vi "FPGAcode4_Test3.vi"() -> ()   [LabVIEW 2015]
uses:
  Limits_In.ctl
  Detector_Cluster.ctl
  <vilib>/Platform/TimedLoop/XDataNode/timing_clust.ctl
  <vilib>/Platform/TimedLoop/XDataNode/nitl_modes.ctl
  <vilib>/Platform/TimedLoop/XDataNode/wakeup.ctl
  Correlations.ctl
  <vilib>/rvi/Emulation/niFpgaGetClockAttributes.vi
  <vilib>/rvi/Emulation/niFpgaSctlEmulationGetInTimedLoop.vi
  <vilib>/rvi/Emulation/niFpgaEmulationReportErrorSimple.vi
  <vilib>/rvi/Emulation/niFpgaProcessEmulError.vi
  <vilib>/rvi/eio/common/nirviEmuTemplateMethod_errors.vi
  <vilib>/rvi/Emulation/niFpgaCriticalErrorInLSC.vi
  <vilib>/eio/EIONode/EIONode.xnode
  <vilib>/Platform/TimedLoop/XDataNode/XDataNode.xnode
  <vilib>/Platform/TimedLoop/XDataNode/XDNodeRunTimeDep.lvlib
panel:
  out "Detectors":T1
  in  "User Trigger?":bool
  in  "User Trigger Distance":fxp<+/-,34,18> format="%.3g"
  out "User Trigger":bool
  in  "Charge Error Factor":fxp<+,32,0>=0.19999999995343387 format="%_2g"
  in  "Threshold Factor":fxp<+/-,32,16>=1.149993896484375 format="%.2g"
  out "DCS 2":bool
  out "DCS 1":bool
  in  "Limits":T2={"High Charge Limit"=4.54747350780585e-13, "Low Charge Limit"=0.0, "High Velocity Limit"=262143.0, "Low Velocity Limit"=0.0, "High Mass Limit"=7.27595761248936e-12, "Low Mass Limit"=0.0, "High Voltage"=2200000.0}
  in  "Calibrate":bool=TRUE
  in  "Armed":bool
  out "Plates":bool
  in  "One Shot":bool
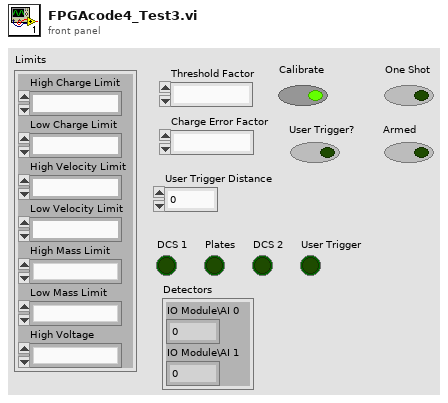
[diagram p1: front panel]
types:
  T1 = cluster{"IO Module\\AI 0":i16, "IO Module\\AI 1":i16}
  T2 = typedef "Limits_In.ctl" = cluster{"High Charge Limit":fxp<+,32,-41>, "Low Charge Limit":fxp<+,32,-41>, "High Velocity Limit":fxp<+,18,18>, "Low Velocity Limit":fxp<+,18,18>, "High Mass Limit":fxp<+/-,33,-36>, "Low Mass Limit":fxp<+/-,33,-36>, "High Voltage":fxp<+,32,22>}
  T3 = typedef "Detector_Cluster.ctl" = cluster{"Det 1":i32, "Det 2":i32}
  T4 = cluster{"Filter 1":T3, "Filter 2":T3, "Filter 3":T3, "Filter 4":T3}
  T5 = cluster{"Distance to PSU":fxp<+/-,32,5>, "Distance to end of PSU":fxp<+/-,32,5>, "Distance to DCS 2":fxp<+/-,32,5>, "Distance to DCS 1":fxp<+/-,32,5>, "Distance to front of LEIL Chamber":fxp<+/-,32,5>}
  T6 = cluster{"Detector Max Speed Count":i32, "Detector Min Speed Count":i32, "Gap Max Speed Count":i32, "Gap Min Speed Count":i32}
  T7 = cluster{"Distance to PSU":fxp<+/-,64,37>, "Distance to end of PSU":fxp<+/-,64,37>, "Distance to DCS 2":fxp<+/-,64,37>, "Distance to DCS 1":fxp<+/-,64,37>, "Distance to front of LEIL Chamber":fxp<+/-,64,37>}
  T8 = cluster{"Filter 1":T3, "Filter 2":T3, "Filter 3":T3, "Filter 4":T3}[]
  T9 = typedef "XDNodeRunTimeDep.lvlib/timing_clust.ctl" = cluster{"Expected End [f-1]":u64, "Actual End [f-1]":u64, "Finished Late? [f-1]":bool, "Expected End [i-1]":u64, "Actual End [i-1]":u64, "Finished Late? [i-1]":bool, "Expected Start [i]":u64, "Actual Start [i]":u64, "Expected Start [f]":u64, "Actual Start [f]":u64, "Source Name":string, "Structure Name":string, "Period":i64, "Deadline":i64, "Offset":i64, "Start":i64, "Priority":i32, "Timeout":i32, "Mode":T10, "Wakeup Reason":T11, "Error":errorcluster, "Source Type":string, "Secondary Source Type":string, "Global End Time":u64, "Global Start Time":u64, "Frame Duration":u64, "Iteration Duration":u64, "Assigned CPU":i32, "I/O Scan Engine Mode":u32}
  T10 = typedef "XDNodeRunTimeDep.lvlib/nitl_modes.ctl" = enum32{"No Change", "Process missed periods, maintain original phase", "Discard missed periods, maintain original phase", "Process missed periods, ignore original phase", "Discard missed periods, ignore original phase"}
  T11 = typedef "XDNodeRunTimeDep.lvlib/wakeup.ctl" = enum32{"Normal", "Aborted", "Asynchronous wakeup", "Timing source error", "Timed loop error", "Timeout"}
  T12 = cluster{"First Detector Count":i32, "Detector Gap Count":i32, "Second Detector Count":i32, "Second Detector Final Count":i32}
  T13 = typedef "Correlations.ctl" = cluster{"First Correlation":i32, "Latest Correlation":i32}
  T14 = cluster{"Distance to PSU":i32, "Distance to end of PSU":i32, "Distance to DCS 2":i32, "Distance to DCS 1":i32, "Distance to front of LEIL Chamber":i32}
  T15 = cluster{"Detectors":cluster{"IO Module\\AI 0":i16, "IO Module\\AI 1":i16}, cluster{"Det 1":i16, "Det 2":i16}, cluster{"Det 1":i16, "Det 2":i16}, cluster{"Det 1":i16, "Det 2":i16}}
  T16 = cluster{cluster{"Det 1":i16, "Det 2":i16}, cluster{"Det 1":i16, "Det 2":i16}, cluster{"Det 1":i16, "Det 2":i16}, cluster{"Det 1":i16, "Det 2":i16}}
  T17 = cluster{"fixed-point type":fxp<+,32,28>, fxp<+/-,64,-6>, fxp<+/-,64,-16>}
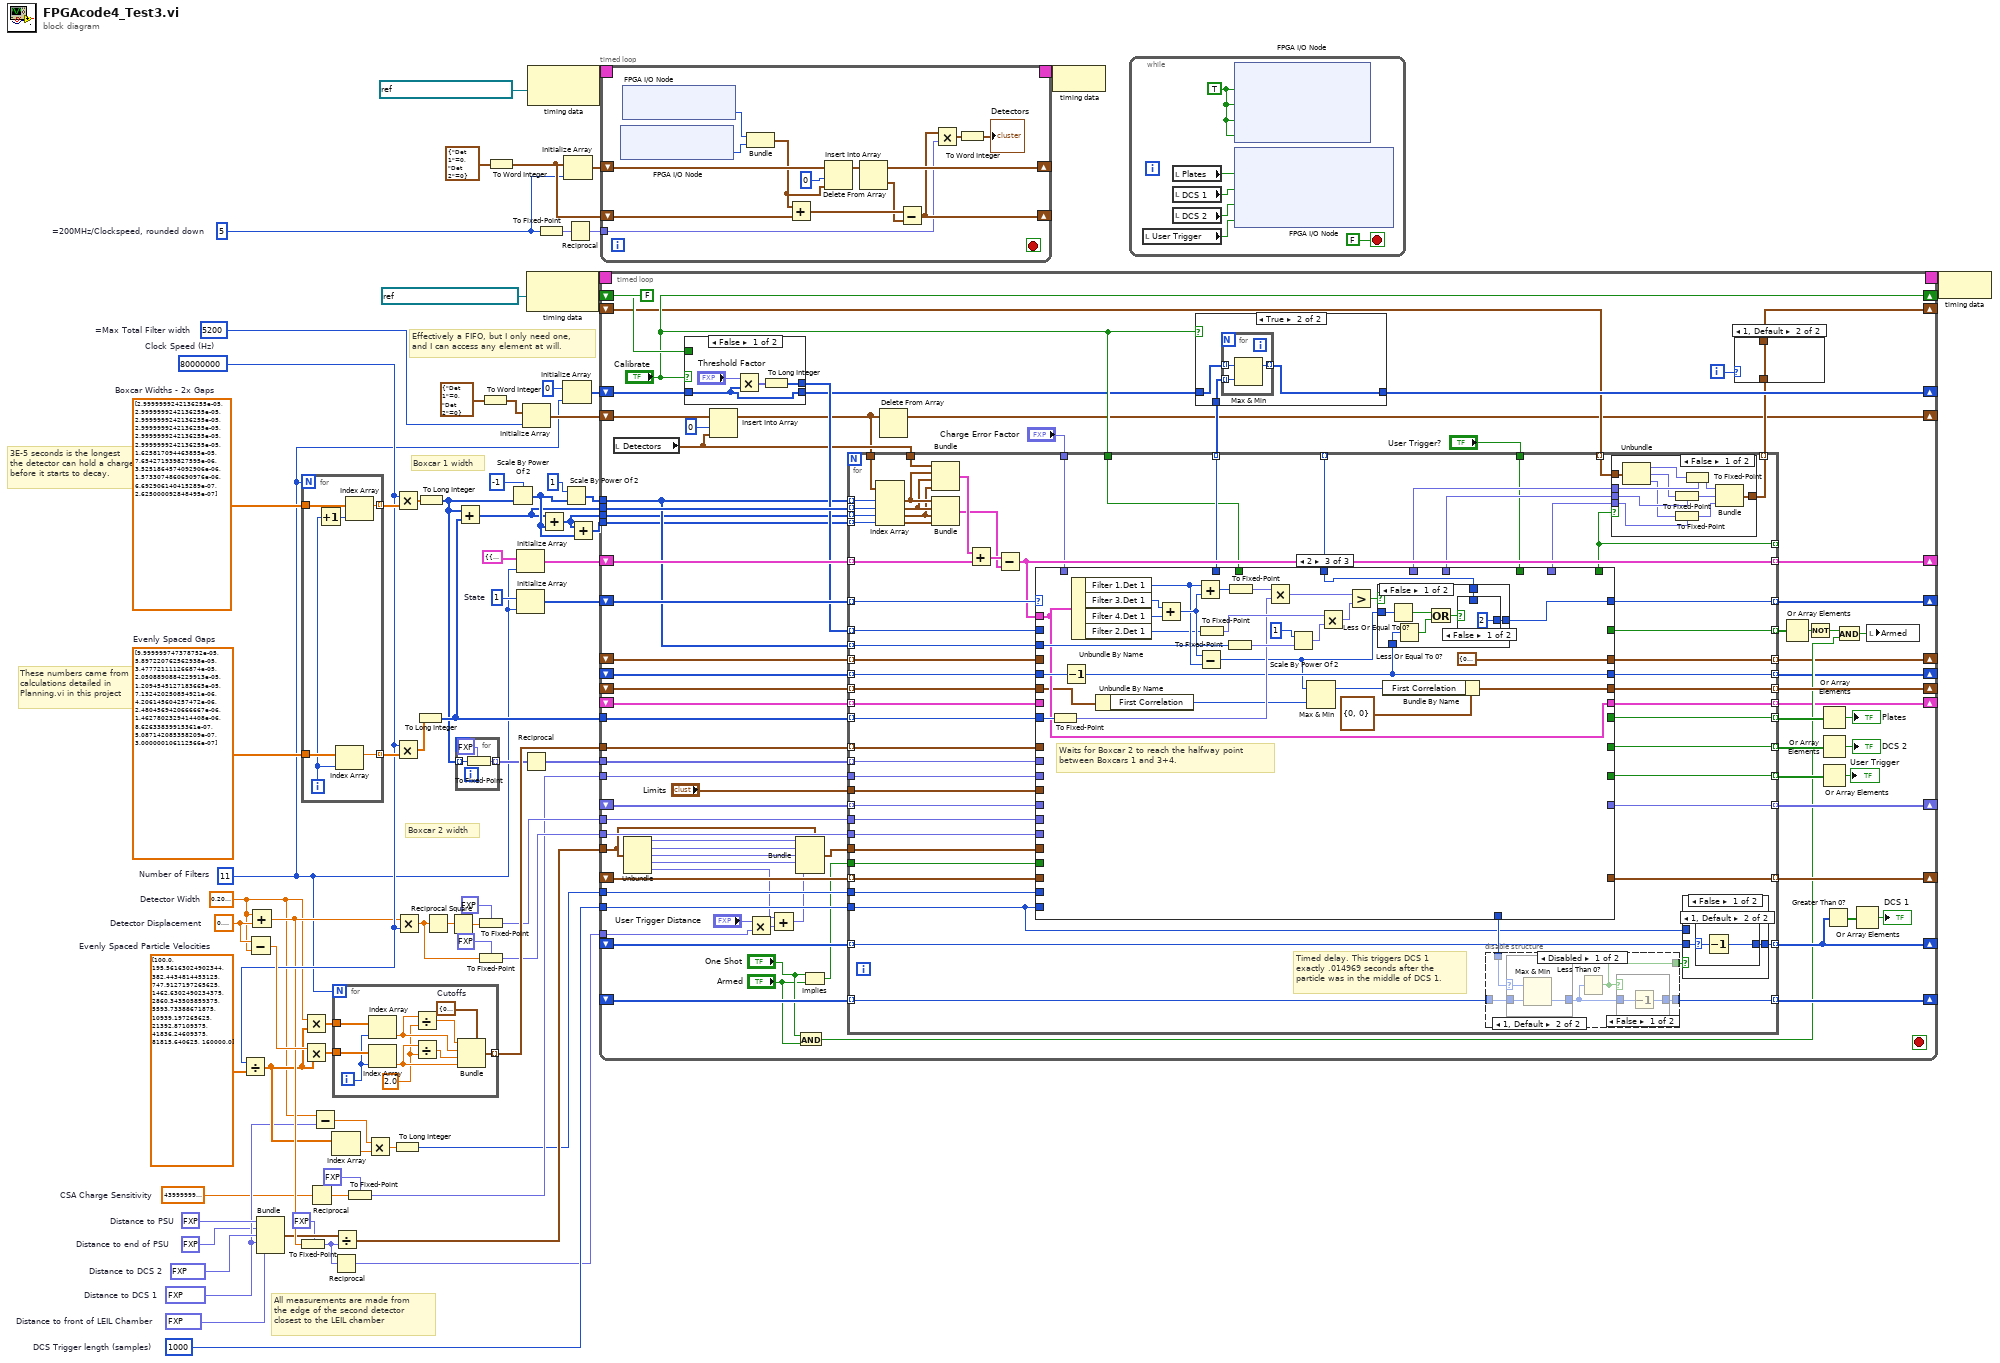
[diagram p0: block diagram]
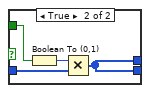
[diagram p3: hidden frame]
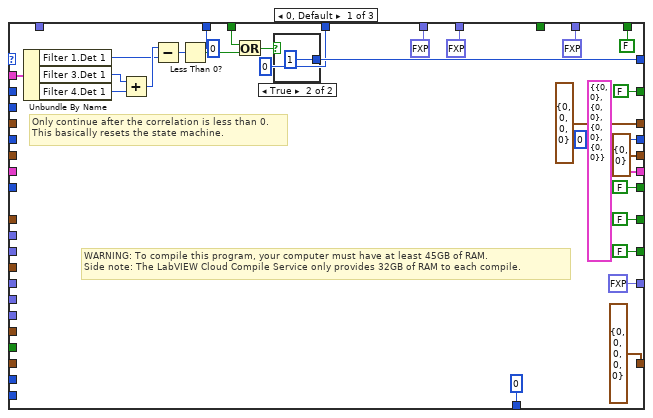
[diagram p5: hidden frame]
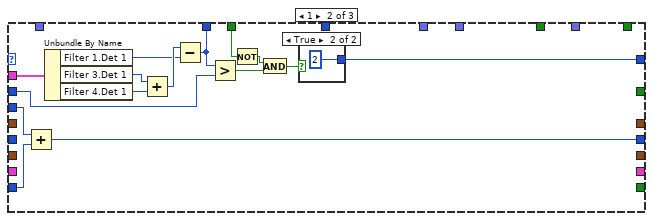
[diagram p7: hidden frame]
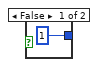
[diagram p8: hidden frame]
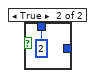
[diagram p9: hidden frame]
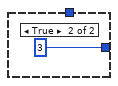
[diagram p10: hidden frame]
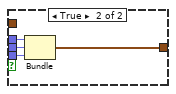
[diagram p11: hidden frame]
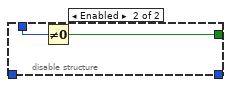
[diagram p16: hidden frame]
diagram:
  w3 = u8 5  # =200MHz/Clockspeed, rounded down
  w10 = 5200  # =Max Total Filter width
  w56 = 80000000  # Clock Speed (Hz)
  w17 = sgl[] [3e-05, 3e-05, 3e-05, 3e-05, 3e-05, 3e-05, 1.6258171e-05, 7.654272e-06, 3.5251865e-06, 1.5733075e-06, 6.692906e-07, 2.625e-07]  # Boxcar Widths - 2x Gaps
  w29 = fxp<+/-,32,5> 4.297679997980595  # Distance to front of LEIL Chamber
  w34 = u16 1000  # DCS Trigger length (samples)
  w39 = fxp<+/-,32,5> -1.3589000031352043  # Distance to DCS 1
  w42 = fxp<+/-,32,5> 2.6162000000476837  # Distance to DCS 2
  w32 = fxp<+/-,32,5> 2.0  # Distance to end of PSU
  w43 = fxp<+/-,32,5> 1.0  # Distance to PSU
  w28 = sgl 4400000000000000.0  # CSA Charge Sensitivity
  w73 = u8 1  # State
  w40 = sgl 0.6  # Detector Displacement
  w68 = sgl[] [0.0001, 5.8972208e-05, 3.477721e-05, 2.050889e-05, 1.2094545e-05, 7.1324203e-06, 4.2061456e-06, 2.480457e-06, 1.4627802e-06, 8.6263384e-07, 5.087142e-07, 3e-07]  # Evenly Spaced Gaps
  w59 = sgl[] [100.0, 195.56163, 382.44348, 747.9127, 1462.6302, 2860.3435, 5593.734, 10939.197, 21392.871, 41836.246, 81815.64, 160000.0]  # Evenly Spaced Particle Velocities
  w35 = sgl 0.21  # Detector Width
  w11 = 11  # Number of Filters
  # "All measurements are made from\nthe edge of the second detector\nclosest to the LEIL chamber"
  # "Effectively a FIFO, but I only need one,\nand I can access any element at will."
  # "Boxcar 2 width"
  # "Boxcar 1 width"
  # "3E-5 seconds is the longest\nthe detector can hold a charge\nbefore it starts to decay."
  # "These numbers came from\ncalculations detailed in\nPlanning.vi in this project"
  n1 = Divide(x=w56, y=w59) -> (x/y=w41:sgl[])
  n2 = Subtract(x=w40, y=w35) -> (x-y=w58:sgl)
  n3 = Add(x=w35, y=w40) -> (x+y=w46:sgl)
  n4 = Bundle("Distance to PSU"=w43, "Distance to end of PSU"=w32, "Distance to DCS 2"=w42, "Distance to DCS 1"=w39, "Distance to front of LEIL Chamber"=w29) -> (w45:T5)  [unwired: 1 in]
  n5 = To Fixed-Point(fixed-point type=fxp<+/-,32,1> 0.0, number=w46) -> (fixed-point=w31:fxp<+/-,32,1>)
  n6 = for {
    N: w11 -> [_]
    tunnel: w68 -> [w83]
    tunnel: [w80] -> w67 mode=indexing
    tunnel: w17 -> [w82]
    tunnel: [w81] -> w66 mode=indexing
    i -> [w79]
    n7 = Increment(x=w79) -> (x+1=w78:i32)
    n8 = Index Array(array=w83, index=w79) -> (element=w80:sgl)
    n9 = Index Array(array=w82, index=w78) -> (element=w81:sgl)
  }
  n10 = Multiply(x=w35, y=w41) -> (x*y=w75:sgl[])
  n11 = Multiply(x=w58, y=w41) -> (x*y=w76:sgl[])
  n12 = Reciprocal(x=w28) -> (1/x=w48:sgl)
  n13 = Subtract(x=w35, y=w39) -> (x-y=w37:sgl)
  n14 = Index Array(array=w41) -> (element=w38:sgl)  [unwired: 1 in]
  n15 = Reciprocal(x=w31) -> (1/x=w30:fxp<+/-,34,33>)
  n16 = for {
    N: w11 -> [_]
    tunnel: w76 -> [w93]
    tunnel: w75 -> [w92]
    tunnel: [w91] -> w70 mode=indexing
    i -> [w90]
    w84 = sgl 2.0 ("y")
    w89 = T6 {"Detector Max Speed Count"=0, "Detector Min Speed Count"=0, "Gap Max Speed Count"=0, "Gap Min Speed Count"=0}  # Cutoffs
    n17 = Index Array(array=w92, index=w90) -> (element=w88:sgl)
    n18 = Index Array(array=w93, index=w90) -> (element=w85:sgl)
    n19 = Divide(x=w88, y=w84) -> (x/y=w87:sgl)
    n20 = Divide(x=w85, y=w84) -> (x/y=w86:sgl)
    n21 = Bundle(cluster=w89, "Detector Max Speed Count"=w87, "Detector Min Speed Count"=w88, "Gap Max Speed Count"=w86, "Gap Min Speed Count"=w85) -> (w91:T6)
  }
  n22 = Divide(x=w45, y=w31) -> (x/y=w44:T7)
  n23 = To Fixed-Point(fixed-point type=fxp<+,32,-49> 0.0, number=w48) -> (fixed-point=w47:fxp<+,32,-49>)
  n24 = Multiply(x=w37, y=w38) -> (x*y=w36:sgl)
  n25 = To Long Integer(number=w36) -> (32bit integer=w33:i32)
  n26 = Multiply(x=w56, y=w66) -> (x*y=w69:sgl[])
  n27 = Multiply(x=w56, y=w67) -> (x*y=w74:sgl[])
  n28 = Multiply(x=w46, y=w56) -> (x*y=w51:sgl)
  n29 = To Long Integer(number=w74) -> (32bit integer=w65:i32[])
  n30 = To Long Integer(number=w69) -> (32bit integer=w22:i32[])
  n31 = Reciprocal(x=w51) -> (1/x=w55:sgl)
  n32 = Square(x=w55) -> (x^2=w54:sgl)
  n33 = Add(x=w22, y=w65) -> (x+y=w18:i32[])
  n34 = for {
    tunnel: w22 -> [w96] mode=indexing
    tunnel: [w95] -> w61 mode=indexing
    n35 = To Fixed-Point(fixed-point type=fxp<+/-,32,32> 0.0, number=w96) -> (fixed-point=w95:fxp<+/-,32,32>)
  }
  n36 = To Fixed-Point(fixed-point type=fxp<+/-,32,-42> 0.0, number=w54) -> (fixed-point=w57:fxp<+/-,32,-42>)
  n37 = To Fixed-Point(fixed-point type=fxp<+,32,28> 0.0, number=w51) -> (fixed-point=w49:fxp<+,32,28>)
  n38 = To Word Integer(number=T3 {"Det 1"=0, "Det 2"=0} ("Detectors")) -> (16bit integer=w64:cluster{"Det 1":i16, "Det 2":i16})
  n39 = To Word Integer(number=T3 {"Det 1"=0, "Det 2"=0} ("Detectors")) -> (16bit integer=w4:cluster{"Det 1":i16, "Det 2":i16})
  n40 = Scale By Power Of 2(n=i16 -1, x=w22) -> (x*2^n=w20:i32[])
  n41 = Initialize Array(T4 {"Filter 1"={"Det 1"=0, "Det 2"=0}, "Filter 2"={"Det 1"=0, "Det 2"=0}, "Filter 3"={"Det 1"=0, "Det 2"=0}, "Filter 4"={"Det 1"=0, "Det 2"=0}} ("cluster"), w11) -> (w71:T8)
  n42 = Initialize Array(w73, w11) -> (w72:u8[])
  n43 = Initialize Array(w64, w10) -> (w77:cluster{"Det 1":i16, "Det 2":i16}[])
  n44 = Reciprocal(x=w61) -> (1/x=w60:fxp<+/-,34,2>[])
  n45 = node-c288(refnum<k21> "40 MHz Onboard Clock" ("Source Name")) -> (w16:T9)
  n46 = node-c288(refnum<k21> "IO Module\\Data Clock" ("Source Name")) -> (w9:T9)
  n47 = To Fixed-Point(number=w3) -> (fixed-point=w2:fxp<+,8,8>)  [unwired: 1 in]
  n48 = Add(x=w18, y=w20) -> (x+y=w21:i32[])
  n49 = Scale By Power Of 2(n=i16 1, x=w20) -> (x*2^n=w25:i32[])
  n50 = Initialize Array(0 ("Thresholds in"), w11) -> (w12:i32[])
  n51 = Initialize Array(w4, w3) -> (w6:cluster{"Det 1":i16, "Det 2":i16}[])
  n52 = Reciprocal(x=w2) -> (1/x=w1:fxp<+,9,1>)
  n53 = Add(x=w21, y=w20) -> (x+y=w19:i32[])
  n54 = timed-loop {
    shift-right: [w97] -> _
    shift-left: w77 -> [w174]
    shift-right: [w106] -> _
    shift-left: w71 -> [w171]
    shift-right: [w100] -> _
    shift-left: w72 -> [w173]
    shift-right: [w107] -> _
    shift-left: _ -> [w172]
    tunnel: w70 -> [w170]
    shift-right: [w169] -> _
    shift-left: _ -> [w168]
    tunnel: w25 -> [w105]
    tunnel: w18 -> [w167]
    tunnel: w65 -> [w166]
    tunnel: w60 -> [w165]
    shift-right: [w164] -> _
    shift-left: _ -> [w163]
    tunnel: w57 -> [w162]
    tunnel: w47 -> [w161]
    tunnel: w49 -> [w160]
    tunnel: w44 -> [w147]
    shift-right: [w159] -> _
    shift-left: _ -> [w158]
    shift-right: [w157] -> _
    shift-left: w12 -> [w156]
    shift-right: ["Calibrate"] -> _
    shift-left: FALSE ("Calibrate") -> [w155]
    tunnel: w34 -> [w154]
    tunnel: w33 -> [w153]
    shift-right: [w151] -> _
    shift-left: _ -> [w152]
    shift-right: [w150] -> _
    shift-left: _ -> [w149]
    tunnel: w30 -> [w148]
    shift-right: [w116] -> _
    shift-left: _ -> [w115]
    shift-right: [w109] -> _
    shift-left: _ -> [w111]
    shift-right: [w104] -> _
    shift-left: _ -> [w103]
    tunnel: w19 -> [w102]
    tunnel: w21 -> [w101]
    timing: w16 -> [_]
    timing-out: [_] -> w15
    i -> [w110]
    stop <- _ stop-if-true
    n55 = local read "Detectors"() -> (w99:T1)
    n56 = Unbundle(w147) -> ("Distance to PSU"=w138:fxp<+/-,64,37>, "Distance to end of PSU"=w137:fxp<+/-,64,37>, "Distance to DCS 2"=w136:fxp<+/-,64,37>, "Distance to DCS 1"=w133:fxp<+/-,64,37>, "Distance to front of LEIL Chamber"=w132:fxp<+/-,64,37>)
    n57 = case shown="False" "Calibrate" {
      tunnel: w156 -> [w177 w183]
      tunnel: [w177 w180] -> w112
      tunnel: w155 -> [_ w182]
      tunnel: [w176 w180] -> w113
      frame False {
        n58 = Multiply(x="Threshold Factor", y=w177) -> (x*y=w178:fxp<+/-,64,48>[])
        n59 = To Long Integer(number=w178) -> (32bit integer=w176:i32[])
      }
      frame True {
        n60 = Boolean To (0,1)(Boolean=w182) -> (0, 1=w181:i16)
        n61 = Multiply(x=w181, y=w183) -> (x*y=w180:i32[])
      }
    }
    n62 = Insert Into Array(array=w174, index=0, new element=w99) -> (w98:cluster{"Det 1":i16, "Det 2":i16}[])
    n63 = Multiply(x="User Trigger Distance", y=w148) -> (x*y=w134:fxp<+/-,64,49>)
    n64 = Add(x=w132, y=w134) -> (x+y=w131:fxp<+/-,64,50>)
    n65 = Bundle(cluster=w147, "Distance to PSU"=w138, "Distance to end of PSU"=w137, "Distance to DCS 2"=w136, "Distance to DCS 1"=w133, "Distance to front of LEIL Chamber"=w131) -> (w135:T7)
    n66 = And(x="One Shot", y="Armed") -> (x .and. y?=w122:bool)
    n67 = Implies(1:"Armed", 2:"One Shot") -> (0:w142:bool)
    n68 = for {
      tunnel: w98 -> [w253]
      tunnel: [w239] -> w106 mode=indexing
      tunnel: w173 -> [w252] mode=indexing
      tunnel: [w251] -> w100 mode=indexing
      tunnel: w113 -> [w194] mode=indexing
      tunnel: [w250] -> w107 mode=indexing
      tunnel: w172 -> [w249] mode=indexing
      tunnel: w171 -> [w243] mode=indexing
      tunnel: w99 -> [w248]
      tunnel: w170 -> [w238] mode=indexing
      tunnel: [w237] -> w169 mode=indexing
      tunnel: w168 -> [w236] mode=indexing
      tunnel: w105 -> [w235] mode=indexing
      tunnel: w167 -> [w192] mode=indexing
      tunnel: w101 -> [w234] mode=indexing
      tunnel: w102 -> [w233] mode=indexing
      tunnel: w105 -> [w198] mode=indexing
      tunnel: w166 -> [w197] mode=indexing
      tunnel: "Charge Error Factor" -> [w232]
      tunnel: [w231] -> _ mode=indexing
      tunnel: w165 -> [w230] mode=indexing
      tunnel: "Limits" -> [w229]
      tunnel: [w228] -> w164 mode=indexing
      tunnel: w163 -> [w227] mode=indexing
      tunnel: w162 -> [w226]
      tunnel: w161 -> [w225]
      tunnel: w160 -> [w224]
      tunnel: w135 -> [w223]
      tunnel: [w222] -> w159 mode=indexing
      tunnel: w158 -> [w221] mode=indexing
      tunnel: [w220] -> w143 mode=indexing
      tunnel: w142 -> [w219]
      tunnel: w154 -> [w216]
      tunnel: w153 -> [w218]
      tunnel: [w215] -> w151 mode=indexing
      tunnel: w152 -> [w214] mode=indexing
      tunnel: [w212] -> w150 mode=indexing
      tunnel: w149 -> [w211] mode=indexing
      tunnel: [w210] -> w130 mode=indexing
      tunnel: [w209] -> w129 mode=indexing
      tunnel: [w208] -> w128 mode=indexing
      tunnel: [w207] -> w125 mode=indexing
      tunnel: "User Trigger?" -> [w203]
      tunnel: w115 -> [w202] mode=indexing
      tunnel: [w201] -> w116 mode=indexing
      tunnel: "Calibrate" -> [w200]
      tunnel: [w196] -> w108 mode=indexing
      tunnel: w111 -> [w199] mode=indexing
      tunnel: [w195] -> _ mode=indexing
      tunnel: [w193] -> w104 mode=indexing
      tunnel: w103 -> [w191] mode=indexing
      # "Timed delay. This triggers DCS 1\nexactly .014969 seconds after the\nparticle was in the middle of DCS 1."
      n69 = Index Array(array=w253, index #1=w235, index #2=w192, index #3=w234, index #4=w233) -> (element #1=w246:cluster{"Det 1":i16, "Det 2":i16}, element #2=w245:cluster{"Det 1":i16, "Det 2":i16}, element #3=w244:cluster{"Det 1":i16, "Det 2":i16}, element #4=w247:cluster{"Det 1":i16, "Det 2":i16})
      n70 = Bundle("Detectors"=w248, w246, w245, w244) -> (w242:T15)  [unwired: 1 in]
      n71 = Bundle(w246, w245, w244, w247) -> (w240:T16)  [unwired: 1 in]
      n72 = Add(x=w242, y=w243) -> (x+y=w241:T4)
      n73 = Subtract(x=w241, y=w240) -> (x-y=w239:T4)
      n74 = case shown="2" w252 {
        tunnel: w194 -> [_ w296 _]
        tunnel: [w279 w294 w326] -> w251
        tunnel: w198 -> [_ w284 w317]
        tunnel: [T12 {"First Detector Count"=0, "Detector Gap Count"=0, "Second Detector Count"=0, "Second Detector Final Count"=0} ("Cutoffs") _ T12 {"First Detector Count"=0, "Detector Gap Count"=0, "Second Detector Count"=0, "Second Detector Final Count"=0} ("Cutoffs")] -> w250
        tunnel: w249 -> [_ _ _]
        tunnel: w191 -> [_ _ w327]
        tunnel: w239 -> [w274 w289 w310]
        tunnel: w238 -> [_ _ _]
        tunnel: w236 -> [_ _ w300]
        tunnel: w197 -> [_ w283 w318]
        tunnel: w232 -> [_ _ _]
        tunnel: [u8 0 ("Det 3") _ w303] -> w231
        tunnel: w230 -> [_ _ _]
        tunnel: w229 -> [_ _ _]
        tunnel: [fxp<+/-,64,-16> 0.0 _ _] -> w228
        tunnel: w227 -> [_ _ _]
        tunnel: w226 -> [_ _ _]
        tunnel: w225 -> [_ _ _]
        tunnel: w224 -> [_ _ _]
        tunnel: w223 -> [_ _ _]
        tunnel: [T14 {"Distance to PSU"=0, "Distance to end of PSU"=0, "Distance to DCS 2"=0, "Distance to DCS 1"=0, "Distance to front of LEIL Chamber"=0} _ _] -> w222
        tunnel: w221 -> [_ _ _]
        tunnel: [0 w288 _] -> w220
        tunnel: w219 -> [_ _ _]
        tunnel: w218 -> [_ _ _]
        tunnel: w216 -> [_ _ _]
        tunnel: [0 _ _] -> w217
        tunnel: [FALSE _ _] -> w210
        tunnel: [FALSE _ _] -> w209
        tunnel: [FALSE _ _] -> w208
        tunnel: [FALSE _ _] -> w207
        tunnel: [fxp<+,32,28> 0.0 ("fixed-point type") _ _] -> w204
        tunnel: [fxp<+/-,64,-16> 0.0 _ _] -> w206
        tunnel: [fxp<+/-,64,-6> 0.0 _ _] -> w205
        tunnel: w203 -> [_ _ _]
        tunnel: [T4 {"Filter 1"={"Det 1"=0, "Det 2"=0}, "Filter 2"={"Det 1"=0, "Det 2"=0}, "Filter 3"={"Det 1"=0, "Det 2"=0}, "Filter 4"={"Det 1"=0, "Det 2"=0}} _ w310] -> w201
        tunnel: w202 -> [_ _ _]
        tunnel: [FALSE ("result") _ _] -> w195
        tunnel: w200 -> [w271 w285 _]
        tunnel: [0 w282 w306] -> w193
        tunnel: [T13 {"First Correlation"=0, "Latest Correlation"=0} ("cluster") _ w312] -> w237
        frame 0, Default {
          # "WARNING: To compile this program, your computer must have at least 45GB of RAM.\nSide note: The LabVIEW Cloud Compile Service only provides 32GB of RAM to each compile."
          # "Only continue after the correlation is less than 0.\nThis basically resets the state machine."
          n75 = Unbundle By Name(w274) -> ("Filter 1.Det 1"=w275:i32, "Filter 3.Det 1"=w276:i32, "Filter 4.Det 1"=w277:i32)
          n76 = Add(x=w276, y=w277) -> (x+y=w278:i32)
          n77 = Subtract(x=w278, y=w275) -> (x-y=w273:i32)
          n78 = Less Than 0?(x=w273) -> (x < 0?=w280:bool)
          n79 = Or(x=w271, y=w280) -> (x .or. y?=w272:bool)
          n80 = case shown="True" w272 {
            tunnel: [_ u8 1 ("Det 3")] -> w279
            frame False {
            }
            frame True {
            }
          }
        }
        frame 1 {
          n81 = Add(x=w284, y=w283) -> (x+y=w282:i32)
          n82 = Unbundle By Name(w289) -> ("Filter 1.Det 1"=w290:i32, "Filter 3.Det 1"=w291:i32, "Filter 4.Det 1"=w292:i32)
          n83 = Add(x=w291, y=w292) -> (x+y=w293:i32)
          n84 = Subtract(x=w293, y=w290) -> (x-y=w288:i32)
          n85 = Greater?(x=w288, y=w296) -> (0:w295:bool)
          n86 = Not(x=w285) -> (.not. x?=w286:bool)
          n87 = And(x=w286, y=w295) -> (x .and. y?=w287:bool)
          n88 = case shown="True" w287 {
            tunnel: [u8 1 ("Det 3") u8 2 ("Det 3")] -> w294
            frame False {
            }
            frame True {
            }
          }
        }
        frame 2 {
          # "Waits for Boxcar 2 to reach the halfway point\nbetween Boxcars 1 and 3+4."
          n89 = To Fixed-Point(number=w318) -> (fixed-point=w307:fxp<+/-,32,32>)  [unwired: 1 in]
          n90 = Decrement(x=w327) -> (x-1=w306:i32)
          n91 = Unbundle By Name(w310) -> ("Filter 1.Det 1"=w320:i32, "Filter 3.Det 1"=w324:i32, "Filter 4.Det 1"=w323:i32, "Filter 2.Det 1"=w314:i32)
          n92 = Unbundle By Name(w300) -> ("First Correlation"=w299:i32)
          n93 = Add(x=w324, y=w323) -> (x+y=w321:i32)
          n94 = Add(x=w320, y=w321) -> (x+y=w325:i32)
          n95 = Subtract(x=w321, y=w320) -> (x-y=w301:i32)
          n96 = To Fixed-Point(number=w314) -> (fixed-point=w309:fxp<+/-,32,32>)  [unwired: 1 in]
          n97 = To Fixed-Point(number=w317) -> (fixed-point=w308:fxp<+/-,32,32>)  [unwired: 1 in]
          n98 = To Fixed-Point(number=w325) -> (fixed-point=w311:fxp<+/-,32,32>)  [unwired: 1 in]
          n99 = Multiply(x=w311, y=w307) -> (x*y=w319:fxp<+/-,64,64>)
          n100 = Scale By Power Of 2(n=i16 1, x=w308) -> (x*2^n=w315:fxp<+/-,32,32>)
          n101 = Max & Min(x=w301, y=w299) -> (max(x,y)=w302:i32)  [unwired: 1 out]
          n102 = Multiply(x=w309, y=w315) -> (x*y=w313:fxp<+/-,64,64>)
          n103 = Greater?(x=w319, y=w313) -> (0:w304:bool)
          n104 = case shown="False" w304 {
            tunnel: [w334 u8 3 ("Det 3")] -> w326
            tunnel: w306 -> [w329 _]
            tunnel: [w333 _] -> w303
            tunnel: w301 -> [w328 _]
            frame False {
              n105 = Less Or Equal To 0?(x=w328) -> (x <= 0?=w331:bool)
              n106 = Less Or Equal To 0?(x=w329) -> (x <= 0?=w330:bool)
              n107 = Or(x=w331, y=w330) -> (x .or. y?=w332:bool)
              n108 = case shown="False" w332 {
                tunnel: [u8 2 ("Det 3") _] -> w334
                tunnel: [_ u8 2 ("Det 3")] -> w333
                frame False {
                }
                frame True {
                }
              }
            }
            frame True {
            }
          }
          n109 = Bundle By Name(cluster=T13 {"First Correlation"=0, "Latest Correlation"=0}, "First Correlation"=w302) -> (w312:T13)
        }
      }
      n110 = disable-structure shown="Disabled" {
        disable-tunnel: w217 -> [w363 w371]
        disable-tunnel: [w359 w370] -> w213
        disable-tunnel: [w361 _] -> w212
        disable-tunnel: w211 -> [w362 _]
        frame Disabled {
          n111 = case shown="1, Default" w363 {
            selector: w363 -> [_ w369]
            tunnel: [w366 w367] -> w360
            tunnel: w362 -> [w366 w368]
            frame 0 {
            }
            frame 1, Default {
              n112 = Max & Min(x=w369, y=w368) -> (min(x,y)=w367:i32)  [unwired: 1 out]
            }
          }
          n113 = Less Than 0?(x=w360) -> (x < 0?=w359:bool)
          n114 = case shown="False" w359 {
            tunnel: w360 -> [w365 _]
            tunnel: [w364 _] -> w361
            frame False {
              n115 = Decrement(x=w365) -> (x-1=w364:i32)
            }
            frame True {
            }
          }
        }
        frame Enabled {
          n116 = Not Equal To 0?(x=w371) -> (x != 0?=w370:bool)
        }
      }
      n117 = case shown="False" w195 {
        tunnel: w206 -> [w343 w350]
        tunnel: w205 -> [w344 w351]
        tunnel: w204 -> [w346 w352]
        tunnel: [w341 w349] -> w196
        tunnel: w199 -> [w348 _]
        frame False {
          n118 = Unbundle(w348) -> ("fixed-point type"=w347:fxp<+,32,28>, w345:fxp<+/-,64,-6>, w342:fxp<+/-,64,-16>)
          n119 = To Fixed-Point(fixed-point type=w344, number=w345) -> (fixed-point=w339:fxp<+/-,64,-6>)
          n120 = To Fixed-Point(fixed-point type=w343, number=w342) -> (fixed-point=w338:fxp<+/-,64,-16>)
          n121 = To Fixed-Point(fixed-point type=w346, number=w347) -> (fixed-point=w340:fxp<+,32,28>)
          n122 = Bundle("fixed-point type"=w340, w339, w338) -> (w341:T17)  [unwired: 1 in]
        }
        frame True {
          n123 = Bundle("fixed-point type"=w352, w351, w350) -> (w349:T17)  [unwired: 1 in]
        }
      }
      n124 = case shown="False" w213 {
        tunnel: w216 -> [_ w358]
        tunnel: [w353 w358] -> w215
        tunnel: w214 -> [w354 _]
        frame False {
          n125 = case shown="1, Default" w354 {
            selector: w354 -> [w355 w357]
            tunnel: [w355 w356] -> w353
            frame 0 {
            }
            frame 1, Default {
              n126 = Decrement(x=w357) -> (x-1=w356:u16)
            }
          }
        }
        frame True {
        }
      }
    }
    n127 = Delete From Array(array=w98) -> (array with subset deleted=w97:cluster{"Det 1":i16, "Det 2":i16}[])  [unwired: 2 in, 1 out]
    n128 = case shown="True" "Calibrate" {
      tunnel: w112 -> [w184 w187]
      tunnel: [w184 w185] -> w157
      tunnel: w143 -> [_ w186]
      frame False {
      }
      frame True {
        n129 = for {
          tunnel: w186 -> [w190] mode=indexing
          tunnel: w187 -> [w189] mode=indexing
          tunnel: [w188] -> w185 mode=indexing
          n130 = Max & Min(x=w189, y=w190) -> (max(x,y)=w188:i32)  [unwired: 1 out]
        }
      }
    }
    n131 = case shown="1, Default" w110 {
      tunnel: [_ w175] -> w109
      tunnel: w108 -> [_ w175]
      frame 0 {
      }
      frame 1, Default {
      }
    }
    n132 = Or Array Elements(Boolean array=w125) -> (logical OR=w119:bool)
    n133 = Not(x=w119) -> (.not. x?=w124:bool)
    n134 = Or Array Elements(Boolean array=w130) -> (logical OR=→"Plates":bool)
    n135 = Or Array Elements(Boolean array=w129) -> (logical OR=→"DCS 2":bool)
    n136 = Or Array Elements(Boolean array=w128) -> (logical OR=→"User Trigger":bool)
    n137 = Greater Than 0?(x=w151) -> (x > 0?=w140:bool[])
    n138 = And(x=w124, y=w122) -> (x .and. y?=w123:bool)
    n139 = Or Array Elements(Boolean array=w140) -> (logical OR=→"DCS 1":bool)
    n140 = local write "Armed"(w123) -> ()
  }
  n141 = timed-loop {
    timing: w9 -> [_]
    timing-out: [_] -> w8
    shift-right: [w382] -> _
    shift-left: w6 -> [w383]
    shift-right: [w377] -> _
    shift-left: w4 -> [w381]
    tunnel: w1 -> [w376]
    stop <- _ stop-if-true
    n142 = xnode "FPGA I/O Node"() -> ("IO Module\\AI 1"=w386:i16)  [unwired: 1 in, 1 out]
    n143 = xnode "FPGA I/O Node"() -> ("IO Module\\AI 0"=w387:i16)  [unwired: 1 in, 1 out]
    n144 = Bundle("IO Module\\AI 0"=w387, "IO Module\\AI 1"=w386) -> (w378:T1)  [unwired: 1 in]
    n145 = Add(x=w378, y=w381) -> (x+y=w380:cluster{i16, i16})
    n146 = Insert Into Array(array=w383, index=0, new element=w378) -> (w384:cluster{"Det 1":i16, "Det 2":i16}[])
    n147 = Delete From Array(array=w384) -> (deleted portion=w379:cluster{"Det 1":i16, "Det 2":i16}, array with subset deleted=w382:cluster{"Det 1":i16, "Det 2":i16}[])  [unwired: 2 in]
    n148 = Subtract(x=w380, y=w379) -> (x-y=w377:cluster{i16, i16})
    n149 = Multiply(x=w377, y=w376) -> (x*y=w375:cluster{fxp<+/-,24,16>, fxp<+/-,24,16>})
    n150 = To Word Integer(number=w375) -> (16bit integer=→"Detectors":cluster{i16, i16})
  }
  n151 = node-c288(w8) -> ()
  n152 = while {
    stop <- FALSE stop-if-true
    w393 = TRUE ("IO Module\\PFI Enable")
    n153 = local read "User Trigger"() -> (w391:bool)
    n154 = local read "Plates"() -> (w394:bool)
    n155 = local read "DCS 1"() -> (w392:bool)
    n156 = local read "DCS 2"() -> (w390:bool)
    n157 = xnode "FPGA I/O Node"("IO Module\\PFI 0 WE"=w393, "IO Module\\PFI 1 WE"=w393, "IO Module\\PFI 2 WE"=w393, "IO Module\\PFI 3 WE"=w393) -> ()  [unwired: 4 in, 4 out]
    n158 = xnode "FPGA I/O Node"("IO Module\\PFI 0 Wr Data"=w394, "IO Module\\PFI 1 Wr Data"=w392, "IO Module\\PFI 2 Wr Data"=w390, "IO Module\\PFI 3 Wr Data"=w391) -> ()  [unwired: 4 in, 4 out]
  }
  n159 = node-c288(w15) -> ()
